vi "chs_sortI.vi"(9 "CHS":T2 {"display" format="%b"}, 10 "Enum":enum16{"CName", "CNO", "ClassI", "ClassII"}(ring)) -> (1 "CH_sort":T1[](array[typedef]) {"CHS"."display" format="%b"})   [LabVIEW 2011]
uses:
  CHS.ctl
  singlechtype.ctl
  chs_sort.ctl
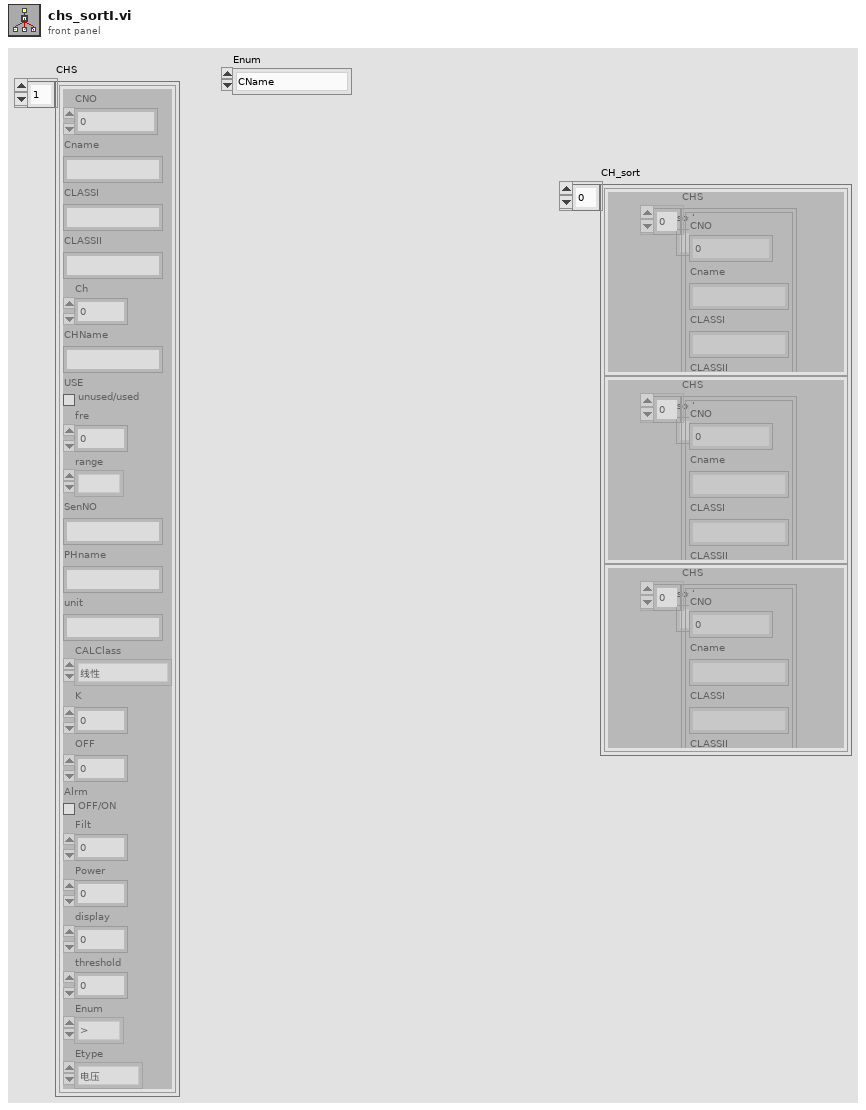
[diagram p1: front panel]
types:
  T1 = typedef "chs_sort.ctl" = cluster{"sort":string, "CHS":T2}
  T2 = typedef "CHS.ctl" = T3[]
  T3 = typedef "singlechtype.ctl" = cluster{"CNO":u8, "Cname":string, "CLASSI":string, "CLASSII":string, "Ch":u8, "CHName":string, "USE":bool, "fre":dbl, "range":enum16{""}, "SenNO":string, "PHname":string, "unit":string, "CALClass":enum8{"线性", "查表", "公式"}, "K":dbl, "OFF":dbl, "Alrm":bool, "Filt":dbl, "Power":u8, "display":u8, "threshold ":dbl, "Enum":enum16{">", ">=", "<", "<=", "<>(在范围内）", "><（在范围外）"}, "Etype":enum16{"电压", "电流", "电阻", "热电偶K", "热电偶T"}}
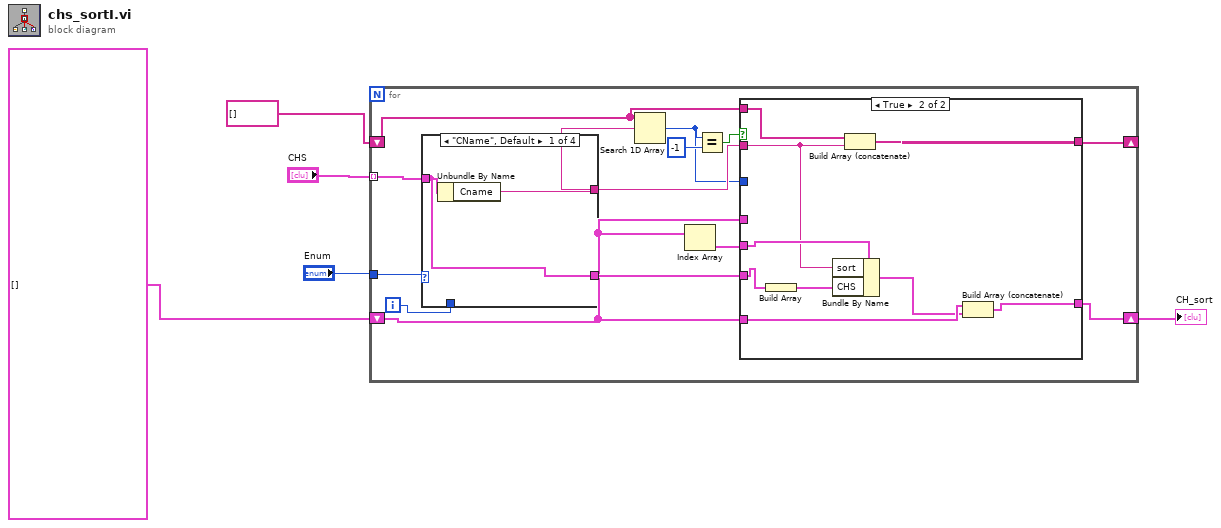
[diagram p0: block diagram]
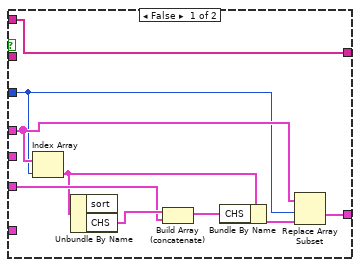
[diagram p2: hidden frame]
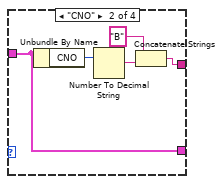
[diagram p3: hidden frame]
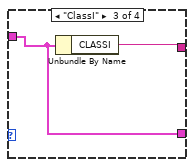
[diagram p4: hidden frame]
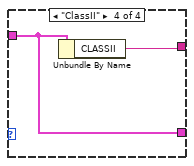
[diagram p5: hidden frame]
diagram:
  n1 = for {
    tunnel: "CHS" -> [w18] mode=indexing
    tunnel: "Enum" -> [w17]
    shift-right: [w10] -> w1
    shift-left: T1[] [] ("CH_sort") -> [w6]
    shift-right: [w12] -> _
    shift-left: string[] [] -> [w14]
    i -> [w16]
    n2 = case shown="\"CName\", Default" w17 {
      tunnel: w18 -> [w37 w42 w44 w46]
      tunnel: [w38 w40 w45 w47] -> w13
      tunnel: w16 -> [_ _ _ _]
      tunnel: [w37 w42 w44 w46] -> w8
      frame "CName", Default {
        n3 = Unbundle By Name(w37) -> ("Cname"=w38:string)
      }
      frame "CNO" {
        n4 = Unbundle By Name(w42) -> ("CNO"=w43:u8)
        n5 = Number To Decimal String(number=w43) -> (decimal integer string=w41:string)  [unwired: 1 in]
        n6 = Concatenate Strings("B" ("string"), w41) -> (w40:string)
      }
      frame "ClassI" {
        n7 = Unbundle By Name(w44) -> ("CLASSI"=w45:string)
      }
      frame "ClassII" {
        n8 = Unbundle By Name(w46) -> ("CLASSII"=w47:string)
      }
    }
    n9 = Search 1D Array(1D array=w14, element=w13) -> (index of element=w7:i32)  [unwired: 1 in]
    n10 = Index Array(array=w6) -> (element=w9:T1)  [unwired: 1 in]
    n11 = Equal?(x=w7, y=-1) -> (x = y?=w11:bool)
    n12 = case shown="True" w11 {
      tunnel: w14 -> [w27 w36]
      tunnel: w13 -> [_ w31]
      tunnel: [w27 w35] -> w12
      tunnel: w6 -> [_ w34]
      tunnel: [w19 w33] -> w10
      tunnel: w9 -> [_ w32]
      tunnel: w8 -> [w25 w30]
      tunnel: w7 -> [w21 _]
      tunnel: w6 -> [w22 _]
      frame False {
        n13 = Index Array(array=w22, index=w21) -> (element=w24:T1)
        n14 = Unbundle By Name(w24) -> ("CHS"=w26:T2)  [unwired: 1 out]
        n15 = Build Array (concatenate)(w26, w25) -> (w23:T2)
        n16 = Bundle By Name(cluster=w24, "CHS"=w23) -> (w20:T1)
        n17 = Replace Array Subset(array=w22, new element=w20, index=w21) -> (w19:T1[])
      }
      frame True {
        n18 = Build Array(w30) -> (w29:T3[])
        n19 = Bundle By Name(cluster=w32, "sort"=w31, "CHS"=w29) -> (w28:T1)
        n20 = Build Array (concatenate)(w36, w31) -> (w35:string[])
        n21 = Build Array (concatenate)(w34, w28) -> (w33:T1[])
      }
    }
  }
  "CH_sort" <- w1
